vi "lnx.vi"(0 "U_ch":i32[](array[numeric]), 1 "Ch":dbl, 2 "i":dbl) -> (3 "x1":dbl, 4 "x2":dbl, 5 "x3":dbl, 6 "x4":dbl)   [LabVIEW 2010]
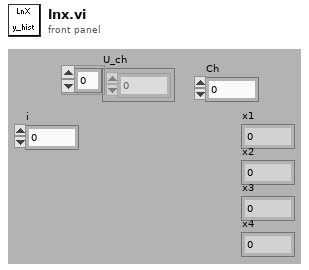
[diagram p1: front panel]
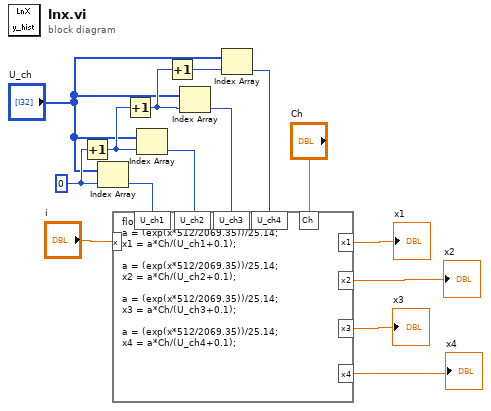
[diagram p0: block diagram]
diagram:
  w12 = 0 ("index")
  n1 = Increment(x=w12) -> (x+1=w10:i32)
  n2 = Index Array(array="U_ch", index=w12) -> (element=w13:i32)
  n3 = Increment(x=w10) -> (x+1=w8:i32)
  n4 = Index Array(array="U_ch", index=w10) -> (element=w11:i32)
  n5 = Increment(x=w8) -> (x+1=w9:i32)
  n6 = Index Array(array="U_ch", index=w8) -> (element=w7:i32)
  n7 = Index Array(array="U_ch", index=w9) -> (element=w6:i32)
  n8 = formula code="float a;\na = (exp(x*512/2069.35))/25.14;\nx1 = a*Ch/(U_ch1+0.1);\n\na = (exp(x*512/2069.35))/25.14;\nx2 = a*Ch/(U_ch2+0.1);\n\na = (exp(x*512/2069.35))/25.14;\nx3 = a*Ch/(U_ch3+0.1);\n\na = (exp(x*512/2069.35))/25.14;\nx4 = a*Ch/(U_ch4+0.1);"("x"="i", "U_ch1"=w13, "Ch"="Ch", "U_ch2"=w11, "U_ch3"=w7, "U_ch4"=w6) -> ("x1"=→"x1":dbl, "x2"=→"x2":dbl, "x3"=→"x3":dbl, "x4"=→"x4":dbl)
